vi "固件升级对话框.vi"() -> ()   [LabVIEW 2016, in "斯坦道CODMn新电路板.lvlib"]
uses:
  <vilib>/Utility/miscctls.llb/LVPointTypeDef.ctl
panel:
  in  "关闭":bool
  in  "固件升级":bool
  in  "固件状态":bool
  out "结果字符串":string
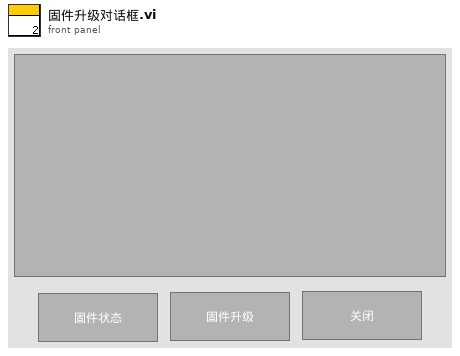
[diagram p1: front panel]
types:
  T1 = typedef "LVPointTypeDef.ctl" = cluster{"Horizontal":i16, "Vertical":i16}
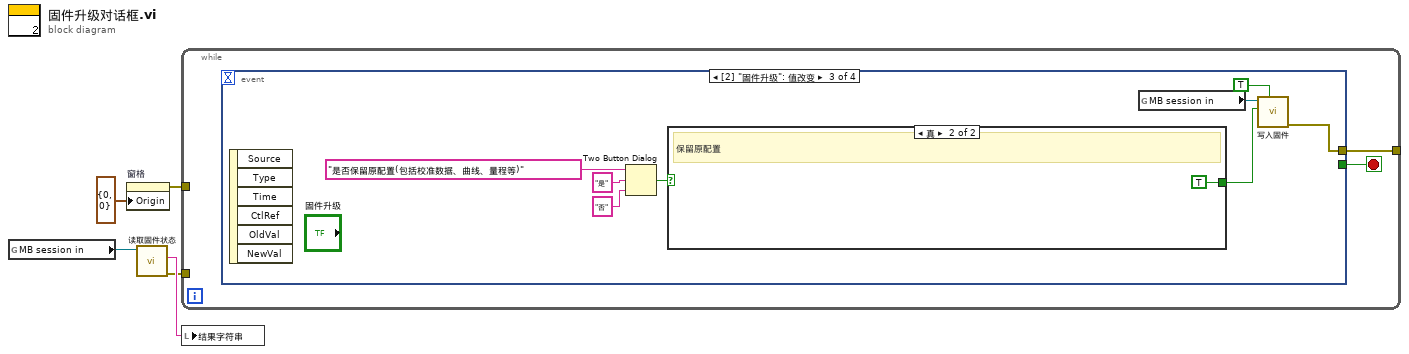
[diagram p0: block diagram]
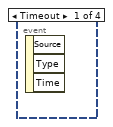
[diagram p2: hidden frame]
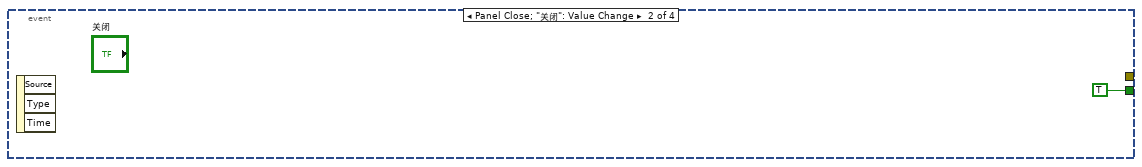
[diagram p3: hidden frame]
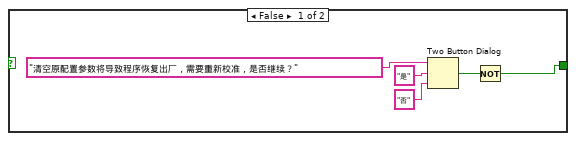
[diagram p4: hidden frame]
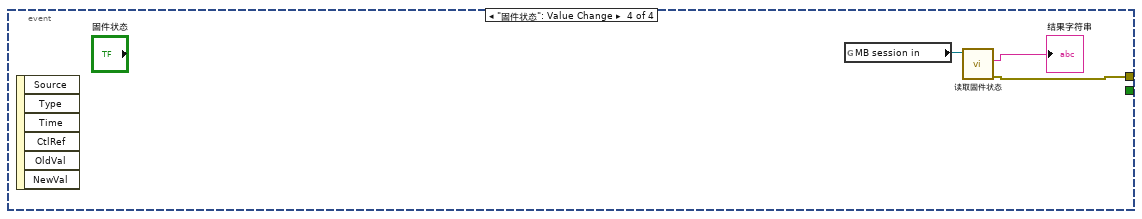
[diagram p5: hidden frame]
diagram:
  n1 = global read "VARCODMn全局变量.vi" "MB session in"() -> (w4:refnum<class "MB_Master.lvclass">)
  n2 = property on="窗格" class="Pane"("Origin"=T1 {"Horizontal"=0, "Vertical"=0} ("原点")) -> (error out=w1:errorcluster)  [unwired: 2 in, 1 out]
  n3 = call "读取固件状态.vi"("MB session in"=w4) -> ("error out"=w2:errorcluster, "结果字符串"=w3:string)  [unwired: 8 in, 1 out]
  n4 = while {
    tunnel: w2 -> [_]
    tunnel: [w6] -> _
    tunnel: w1 -> [_]
    stop <- w7 stop-if-true
    n5 = event shown="[2] \"固件升级\": 值改变" {
      selector: _ -> [_ _ _ _]
      dyn-events: _ -> [_ _ _ _]
      timeout: _ -> [_ _ _ _]
      tunnel: [_ TRUE _ _] -> w7
      tunnel: [_ _ w15 w23] -> w6
      event Timeout {
        n6 = event-data() -> ()  [unwired: 1 in, 3 out]
      }
      event Panel Close; "关闭": Value Change {
        n7 = event-data() -> ()  [unwired: 1 in, 3 out]
      }
      event "固件升级": Value Change {
        n8 = event-data() -> ()  [unwired: 1 in, 6 out]
        n9 = Two Button Dialog(message="是否保留原配置(包括校准数据、曲线、量程等)" ("消息"), 1:"否" ("F按钮名称（“取消”）"), 2:"是" ("T按钮名称（“确定”）")) -> (T button?=w11:bool)
        n10 = case shown="真" w11 {
          tunnel: [w17 TRUE] -> w10
          frame False {
            n11 = Two Button Dialog(message="清空原配置参数将导致程序恢复出厂，需要重新校准，是否继续？" ("消息"), 1:"否" ("F按钮名称（“取消”）"), 2:"是" ("T按钮名称（“确定”）")) -> (T button?=w21:bool)
            n12 = Not(x=w21) -> (.not. x?=w17:bool)
          }
          frame True {
            # "保留原配置"
          }
        }
        n13 = global read "VARCODMn全局变量.vi" "MB session in"() -> (w16:refnum<class "MB_Master.lvclass">)
        n14 = call "写入固件.vi"("路径对话框"=TRUE, "保留原配置"=w10, "MB session in"=w16) -> ("error out"=w15:errorcluster)  [unwired: 7 in, 1 out]
      }
      event "固件状态": Value Change {
        n15 = event-data() -> ()  [unwired: 1 in, 6 out]
        n16 = global read "VARCODMn全局变量.vi" "MB session in"() -> (w24:refnum<class "MB_Master.lvclass">)
        n17 = call "读取固件状态.vi"("MB session in"=w24) -> ("error out"=w23:errorcluster, "结果字符串"=→"结果字符串":string)  [unwired: 8 in, 1 out]
      }
    }
  }
  n18 = local write "结果字符串"(w3) -> ()
